vi "全局 1.vi"() -> ()   [LabVIEW 2018]
panel:
  in  "选项卡控件":enum32{"系统", "PLC", "VISON"}(tab)
  out "产品名称0":string
  out "物料编号4":string
  out "物料编号3":string
  out "产品名称2":string
  in  "系统时间":timestamp
  out "物料编号2":string
  out "机台编号":string
  out "物料编号1":string
  out "产线编号":string
  out "Login PW":dbl[](array[numeric])=[12.34, -43.21] format="%.2f"
  out "Login":i32
  out "CCIEFB Slave IP":string="192.168.2.100"
  out "ROBOT PORT":u16 format="%08x"
  out "ROBOT IP":string
  out "PLC PORT":u16 format="%08x"
  out "PLC IP":string
  out "ini文件":path
  out "产品名称1":string
  out "Exit":bool
  out "检测序号":u16
  out "PLC结果":T1
  out "PLC状态":T2
  out "力":sgl[](array[numeric]) format="%.4f"
  out "检测步骤":T3
  out "PLC检测值":T4 {"3#LED电压" format="%.2f"; "3#LED电流" format="%.2f"; "3#风门开电压" format="%.2f"; "3#风门闭电压" format="%.2f"; "3#稳定压力" format="%.1f"; "3#当前压力" format="%.1f"; "3#稳定泄漏量" format="%.2f"; "3#当前泄漏量" format="%.2f"; "2#LED电压" format="%.2f"; "2#LED电流" format="%.2f"; "2#风门开电压" format="%.2f"; "2#风门闭电压" format="%.2f"; "2#稳定压力" format="%.1f"; "2#当前压力" format="%.1f"; "2#稳定泄漏量" format="%.2f"; "2#当前泄漏量" format="%.2f"; "1#LED电压" format="%.2f"; "1#LED电流" format="%.2f"; "1#风门开电压" format="%.2f"; "1#风门闭电压" format="%.2f"; "1#稳定压力" format="%.1f"; "1#当前压力" format="%.1f"; "1#稳定泄漏量" format="%.2f"; "1#当前泄漏量" format="%.2f"}
  out "高低配":i16
  out "PLC检测参数":T5 {"INV快速变化量" format="%.2f"; "INV慢速变化量" format="%.2f"; "INV变化周期" format="%.1f"; "INV初始频率" format="%.2f"; "伺服速度" format="%.1f"; "气压稳定时间" format="%.1f"; "LED电流下限" format="%.2f"; "LED电流上限" format="%.2f"; "风门开电压下限" format="%.2f"; "风门开电压上限" format="%.2f"; "风门闭电压下限" format="%.2f"; "风门闭电压上限" format="%.2f"; "压力下限" format="%.1f"; "压力上限" format="%.1f"; "泄漏量上限" format="%.2f"; "轮盘预压力" format="%.1f"}
  out "PC状态":cluster{"PLC就绪":bool, "空动作中":bool}
  out "3#视觉检测":u16[](array[numeric])
  out "2#视觉检测":u16[](array[numeric])
  out "1#视觉检测":u16[](array[numeric])
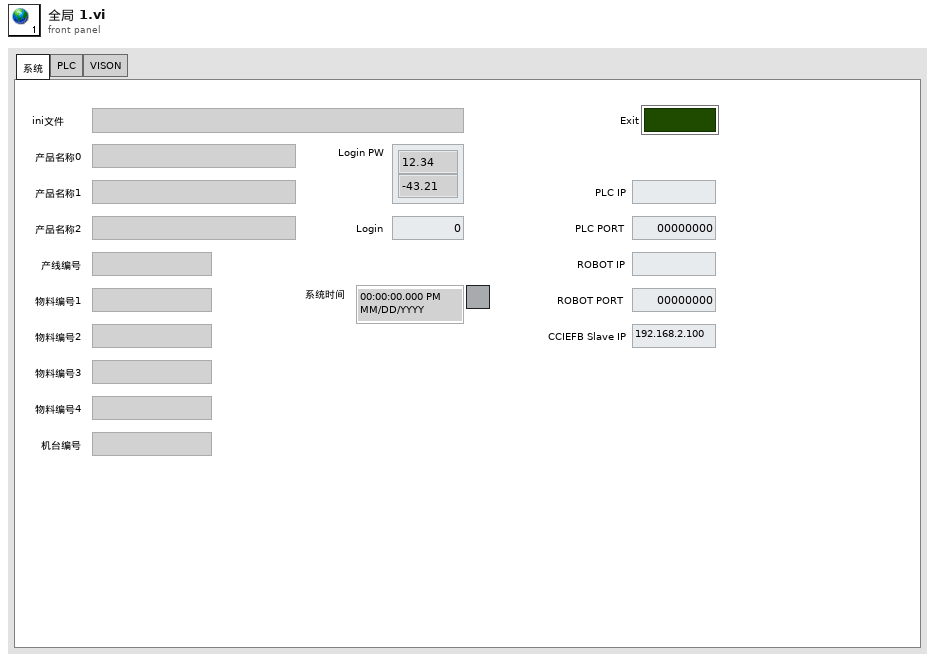
[diagram p1: front panel]
types:
  T1 = cluster{"1#泄漏量":bool, "1#风门闭电压":bool, "1#风门开电压":bool, "1#LED电压":bool, "1#LED电流":bool, "外观结果":bool, "2#泄漏量":bool, "2#风门闭电压":bool, "2#风门开电压":bool, "2#LED电压":bool, "2#LED电流":bool, "3#泄漏量":bool, "3#风门闭电压":bool, "3#风门开电压":bool, "3#LED电压":bool, "3#LED电流":bool}
  T2 = cluster{"PLC就绪":bool, "ROBOT就绪":bool, "空动作":bool, "检测NG":bool, "检测结束":bool, "检测开始":bool, "初始化脉冲":bool, "1#检测NG":bool, "2#检测NG":bool, "3#检测NG":bool}
  T3 = cluster{"泄漏量":bool, "风门开闭电检":bool, "LED电检":bool, "外观检测":bool, "1#轮盘关开":bool, "1#轮盘关开锁":bool, "1#轮盘开关":bool, "1#轮盘开关锁":bool, "1#拨钮左右":bool, "1#拨钮右左":bool, "1#拨钮上下":bool, "1#拨钮下上":bool, "2#轮盘关开":bool, "2#轮盘关开锁":bool, "2#轮盘开关":bool, "2#轮盘开关锁":bool, "2#拨钮左右":bool, "2#拨钮右左":bool, "2#拨钮上下":bool, "2#拨钮下上":bool, "3#轮盘关开":bool, "3#轮盘关开锁":bool, "3#轮盘开关":bool, "3#轮盘开关锁":bool, "3#拨钮左右":bool, "3#拨钮右左":bool, "3#拨钮上下":bool, "3#拨钮下上":bool}
  T4 = cluster{"1#当前泄漏量":sgl, "1#稳定泄漏量":sgl, "1#当前压力":sgl, "1#稳定压力":sgl, "1#风门闭电压":sgl, "1#风门开电压":sgl, "1#LED电流":sgl, "1#LED电压":sgl, "2#当前泄漏量":sgl, "2#稳定泄漏量":sgl, "2#当前压力":sgl, "2#稳定压力":sgl, "2#风门闭电压":sgl, "2#风门开电压":sgl, "2#LED电流":sgl, "2#LED电压":sgl, "3#当前泄漏量":sgl, "3#稳定泄漏量":sgl, "3#当前压力":sgl, "3#稳定压力":sgl, "3#风门闭电压":sgl, "3#风门开电压":sgl, "3#LED电流":sgl, "3#LED电压":sgl}
  T5 = cluster{"轮盘预压力":sgl, "泄漏量上限":sgl, "压力上限":sgl, "压力下限":sgl, "风门闭电压上限":sgl, "风门闭电压下限":sgl, "风门开电压上限":sgl, "风门开电压下限":sgl, "LED电流上限":sgl, "LED电流下限":sgl, "气压稳定时间":sgl, "伺服速度":sgl, "INV初始频率":sgl, "INV变化周期":sgl, "INV慢速变化量":sgl, "INV快速变化量":sgl}
diagram:
